vi "SingleImgProcess.vi"(10 "Process List":string[][](array[string]), 11 "Refnum in":T1) -> (0 "error out":errorcluster, 3 "ImgOut":T1)   [LabVIEW 2019]
uses:
  <vilib>/vision/Image Controls.llb/IMAQ Image.ctl
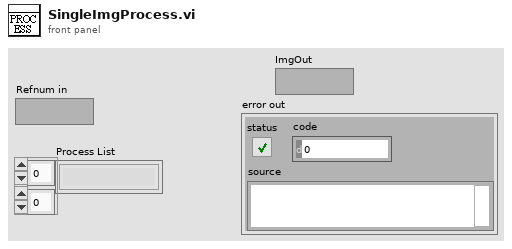
[diagram p1: front panel]
types:
  T1 = typedef "IMAQ Image.ctl" = refnum<image>
  T2 = typedef "Image Type" = u32
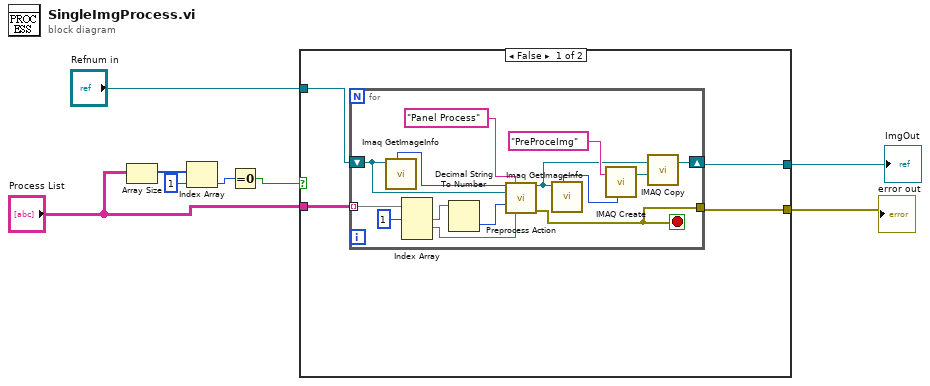
[diagram p0: block diagram]
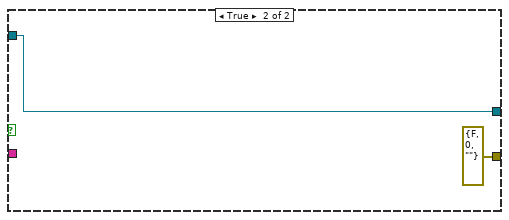
[diagram p2: hidden frame]
diagram:
  n1 = Array Size(array="Process List") -> (size(s)=w4:i32[])
  n2 = Index Array(array=w4, index=1) -> (element=w2:i32)
  n3 = Equal To 0?(x=w2) -> (x = 0?=w1:bool)
  n4 = case shown="False" w1 {
    tunnel: "Refnum in" -> [w12 w28]
    tunnel: [w11 w28] -> w7
    tunnel: [w10 errorcluster {"status"=FALSE, "code"=0, "source"=""} ("error out")] -> w6
    tunnel: "Process List" -> [w9 _]
    frame False {
      n5 = for {
        tunnel: w9 -> [w26] mode=indexing
        shift-right: [w17] -> w11
        shift-left: w12 -> [w23]
        tunnel: [w14] -> w10
        stop <- w14 stop-if-true
        n6 = call "Imaq GetImageInfo"("Image"=w23) -> ("Image Type"=w22:T2)  [unwired: 3 in, 7 out]
        n7 = Index Array(array=w26, index #1=1 ("index")) -> (element #1=w24:string, element #2=w13:string)  [unwired: 2 in, 1 out]
        n8 = Decimal String To Number(string=w24) -> (number=w15:i32)  [unwired: 2 in, 1 out]
        n9 = call "Preprocess Action.vi"("Image Type"=w22, "Image Dust"="Panel Process", "ImageSorce"=w23, "PreProcess"=w15, "Data"=w13) -> ("Refnum out"=w19:T1, "error out"=w14:errorcluster)  [unwired: 9 in]
        n10 = call "Imaq GetImageInfo"("Image"=w19) -> ("Image Type"=w16:T2)  [unwired: 3 in, 7 out]
        n11 = call "IMAQ Create"("Image Name"="PreProceImg", "Image Type"=w16) -> ("New Image"=w18:T1)  [unwired: 3 in, 1 out]
        n12 = call "IMAQ Copy"("Image Dst"=w18, "Image Src"=w19) -> ("Image Dst Out"=w17:T1)  [unwired: 4 in, 1 out]
      }
    }
    frame True {
    }
  }
  "ImgOut" <- w7
  "error out" <- w6
